vi "Calibration_Quadruple_Save.vi"(0 "Data":T2 {"Flush Size" min=1; "Dispense Speed" min=1; "Rectangle 2"."Rotation" format="%.2f"; "Rectangle 2"."Left" scale=0.0..1024.0; "Rectangle 2"."Right" scale=0.0..1024.0; "Rectangle 1"."Rotation" format="%.2f"; "Rectangle 1"."Left" scale=0.0..1024.0; "Rectangle 1"."Right" scale=0.0..1024.0; "Max Framerate" min=1; "Overload threshold" min=1; "Image Save Queue Size" min=1; "Image Process Queue Size" min=1; "Empty start" min=1; "Sample size threshold" min=1; "Framerate" min=1; "Light intensity" scale=0.0..100.0}, 5 "Img1":T1, 7 "Img2":T1, 9 "Path1":string, 11 "Path2":string) -> (4 "Cal1":path, 6 "Cal2":path, 10 "Img1 out":T1, 15 "Img2 out":T1)   [LabVIEW 2020]
uses:
  <vilib>/vision/Image Controls.llb/IMAQ Image.ctl
  controls/Data.ctl
  <vilib>/userDefined/High Color/IMAQdx.ctl
panel:
  out "error out 4":errorcluster
  out "error out 3":errorcluster
  out "error out 2":errorcluster
  out "error out":errorcluster
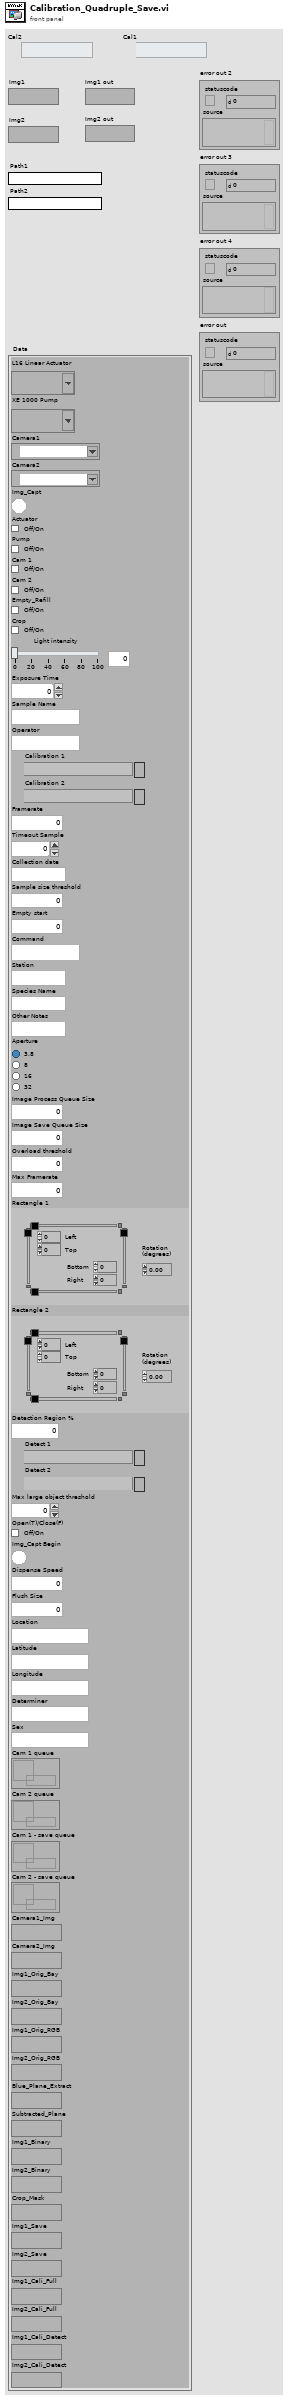
[diagram p1: front panel]
types:
  T1 = typedef "IMAQ Image.ctl" = refnum<image>
  T2 = typedef "Data.ctl" = cluster{"L16 Linear Actuator":refnum<visa-resource-name>, "XE 1000 Pump":refnum<visa-resource-name>, "Camera1":T3, "Camera2":T3, "Img_Capt":bool, "Actuator":bool, "Pump":bool, "Cam 1":bool, "Cam 2":bool, "Empty_Refill":bool, "Crop":bool, "Light intensity":i32, "Exposure Time":dbl, "Sample Name":string, "Operator":string, "Calibration 1":path, "Calibration 2":path, "Framerate":i32, "Timeout Sample":i32, "Collection date":string, "Sample size threshold":i32, "Empty start":u32, "Command":string, "Station":string, "Species Name":string, "Other Notes":string, "Aperture":enum32{"Item 0", "Item 1", "Item 2", "Item 3"}, "Image Process Queue Size":i32, "Image Save Queue Size":i32, "Overload threshold":i32, "Max Framerate":i32, "Rectangle 1":T4, "Rectangle 2":T4, "Detection Region %":dbl, "Detect 1":path, "Detect 2":path, "Max large object threshold":i32, "Open(T)/Close(F)":bool, "Img_Capt Begin":bool, "Dispense Speed":i32, "Flush Size":i32, "Location":string, "Latitude":string, "Longitude":string, "Determiner":string, "Sex":string, "Cam 1 queue":refnum<queue>, "Cam 2 queue":refnum<queue>, "Cam 1 - save queue":refnum<queue>, "Cam 2 - save queue":refnum<queue>, "Camera1_Img":T1, "Camera2_Img":T1, "Img1_Orig_Bay":T1, "Img2_Orig_Bay":T1, "Img1_Orig_RGB":T1, "Img2_Orig_RGB":T1, "Blue_Plane_Extract":T1, "Subtracted_Plane":T1, "Img1_Binary":T1, "Img2_Binary":T1, "Crop_Mask":T1, "Img1_Save":T1, "Img2_Save":T1, "Img1_Cali_Full":T1, "Img2_Cali_Full":T1, "Img1_Cali_Detect":T1, "Img2_Cali_Detect":T1}
  T3 = typedef "IMAQdx.ctl" = refnum<k21>
  T4 = typedef "IMAQ Rectangle" = cluster{"Left":i32, "Top":i32, "Right":i32, "Bottom":i32, "Rotation":dbl}
  T5 = cluster{"Pattern":i32, "Algorithm":i32, "Red Gain":dbl, "Green Gain":dbl, "Blue Gain":dbl}
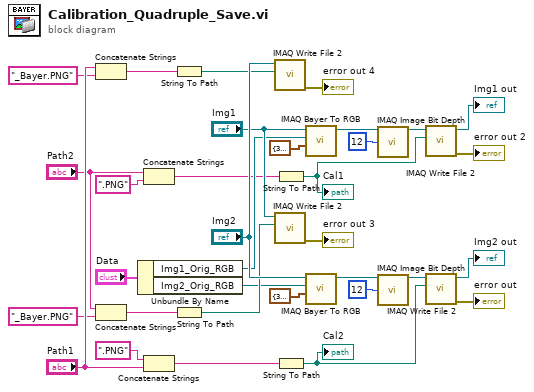
[diagram p0: block diagram]
diagram:
  n1 = Concatenate Strings("Path1", "_Bayer.PNG" ("string")) -> (w30:string)
  n2 = Concatenate Strings("Path2", "_Bayer.PNG" ("string")) -> (w21:string)
  n3 = Unbundle By Name("Data") -> ("Img1_Orig_RGB"=w18:T1, "Img2_Orig_RGB"=w20:T1)
  n4 = Concatenate Strings("Path2", ".PNG" ("string")) -> (w15:string)
  n5 = Concatenate Strings(".PNG" ("string"), "Path1") -> (w17:string)
  n6 = String To Path(string=w30) -> (path=w32:path)
  n7 = String To Path(string=w21) -> (path=w26:path)
  n8 = call-poly "IMAQ Write File 2"("File Path"=w32, "Image"="Img2") -> ("error out"=→"error out 4":errorcluster)  [unwired: 8 in, 1 out]
  n9 = call-poly "IMAQ Write File 2"("File Path"=w26, "Image"="Img1") -> ("error out"=→"error out 3":errorcluster)  [unwired: 8 in, 1 out]
  n10 = String To Path(string=w15) -> (path=w10:path)
  "Cal1" <- w10
  n11 = String To Path(string=w17) -> (path=w7:path)
  "Cal2" <- w7
  n12 = call "IMAQ Bayer To RGB"("Bayer Parameters"=T5 {"Pattern"=3, "Algorithm"=0, "Red Gain"=1.0, "Green Gain"=1.0, "Blue Gain"=1.0}, "Image Dst"=w18, "Image Src"="Img1") -> ("Image Dst Out"=w2:T1)  [unwired: 7 in, 1 out]
  n13 = call "IMAQ Bayer To RGB"("Bayer Parameters"=T5 {"Pattern"=3, "Algorithm"=0, "Red Gain"=1.0, "Green Gain"=1.0, "Blue Gain"=1.0}, "Image Dst"=w20, "Image Src"="Img2") -> ("Image Dst Out"=w5:T1)  [unwired: 7 in, 1 out]
  n14 = call "IMAQ Image Bit Depth"("Image"=w2, "Bit Depth (0)"=u32 12) -> ("Image Out"=w1:T1)  [unwired: 11 in, 2 out]
  n15 = call "IMAQ Image Bit Depth"("Image"=w5, "Bit Depth (0)"=u32 12) -> ("Image Out"=w4:T1)  [unwired: 11 in, 2 out]
  n16 = call-poly "IMAQ Write File 2"("File Path"=w10, "Image"=w1) -> ("error out"=→"error out 2":errorcluster, "Image Out (duplicate)"=→"Img1 out":T1)  [unwired: 8 in]
  n17 = call-poly "IMAQ Write File 2"("File Path"=w7, "Image"=w4) -> ("error out"=→"error out":errorcluster, "Image Out (duplicate)"=→"Img2 out":T1)  [unwired: 8 in]
